vi "getCurrentTimeInMilliseconds.vi"() -> ()   [LabVIEW 2016]
panel:
  out "decimal integer string":string
  out "time":dbl
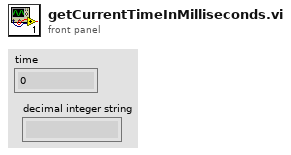
[diagram p1: front panel]
types:
  T1 = typedef "LVDateTimeRec.ctl" = cluster{"fractional second":dbl, "second":i32, "minute":i32, "hour":i32, "day of month":i32, "month":i32, "year":i32, "day of week":i32, "day of year":i32, "DST":i32}
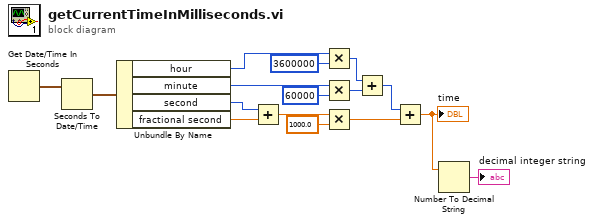
[diagram p0: block diagram]
diagram:
  n1 = Get Date/Time In Seconds() -> (seconds since 1Jan1904=w16:timestamp)
  n2 = Seconds To Date/Time(time stamp (now)=w16) -> (date time rec=w15:T1)  [unwired: 1 in]
  n3 = Unbundle By Name(w15) -> ("hour"=w14:i32, "minute"=w12:i32, "second"=w10:i32, "fractional second"=w9:dbl)
  n4 = Add(x=w10, y=w9) -> (x+y=w8:dbl)
  n5 = Multiply(x=w14, y=3600000) -> (x*y=w6:i32)
  n6 = Multiply(x=w12, y=60000) -> (x*y=w5:i32)
  n7 = Multiply(x=w8, y=1000.0) -> (x*y=w3:dbl)
  n8 = Add(x=w6, y=w5) -> (x+y=w4:i32)
  n9 = Add(x=w4, y=w3) -> (x+y=w2:dbl)
  "time" <- w2
  n10 = Number To Decimal String(number=w2) -> (decimal integer string=→"decimal integer string":string)  [unwired: 1 in]
